vi "CAPTH-Update History.vi"(0 "State in":T1, 7 "Properties":T4, 9 "Ntries":i32) -> (4 "State out":T1)   [LabVIEW 2020]
uses:
  Typedefs/CAPTH-Analysis Data Properties.ctl
  Typedefs/CAPTH-Analysis State.ctl
  Typedefs/CAPTH-History.ctl
  Typedefs/CAPTH-StimCon.ctl
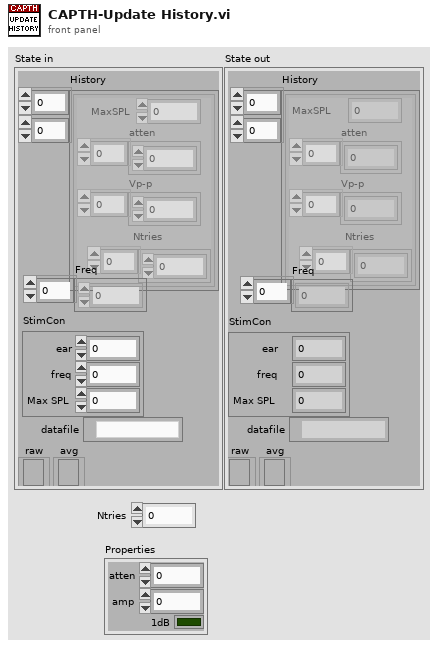
[diagram p1: front panel]
types:
  T1 = typedef "CAPTH-Analysis State.ctl" = cluster{"History":T2, "Freq":dbl[], "StimCon":T3, "datafile":path, "raw":refnum<file>, "avg":refnum<file>}
  T2 = typedef "CAPTH-History.ctl" = cluster{"MaxSPL":dbl, "atten":dbl[], "Vp-p":dbl[], "Ntries":i32[]}[][]
  T3 = typedef "CAPTH-StimCon.ctl" = cluster{"ear":i32, "freq":i32, "Max SPL":dbl}
  T4 = typedef "CAPTH-Analysis Data Properties.ctl" = cluster{"atten":dbl, "amp":dbl, "1dB":bool}
  T5 = cluster{"MaxSPL":dbl, "atten":dbl[], "Vp-p":dbl[], "Ntries":i32[]}
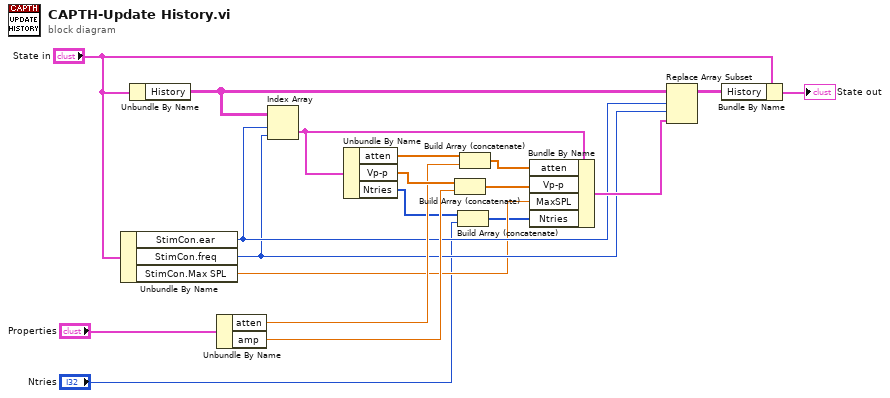
[diagram p0: block diagram]
diagram:
  n1 = Unbundle By Name("State in") -> ("StimCon.ear"=w9:i32, "StimCon.freq"=w8:i32, "StimCon.Max SPL"=w4:dbl)
  n2 = Unbundle By Name("State in") -> ("History"=w11:T2)
  n3 = Unbundle By Name("Properties") -> ("atten"=w16:dbl, "amp"=w15:dbl)
  n4 = Index Array(array=w11, index (row)=w9, index (col)=w8) -> (element=w14:T5)
  n5 = Unbundle By Name(w14) -> ("atten"=w19:dbl[], "Vp-p"=w18:dbl[], "Ntries"=w3:i32[])
  n6 = Build Array (concatenate)(w18, w15) -> (w12:dbl[])
  n7 = Build Array (concatenate)(w3, "Ntries") -> (w1:i32[])
  n8 = Build Array (concatenate)(w19, w16) -> (w13:dbl[])
  n9 = Bundle By Name(cluster=w14, "atten"=w13, "Vp-p"=w12, "MaxSPL"=w4, "Ntries"=w1) -> (w10:T5)
  n10 = Replace Array Subset(array=w11, new element=w10, index (row)=w9, index (col)=w8) -> (w6:T2)
  n11 = Bundle By Name(cluster="State in", "History"=w6) -> (→"State out":T1)
